vi "create Cell.vi"(8 "error in (no error)":errorcluster, 9 "Column":i32, 10 "Row":i32, 11 "Cell in":refnum<class "Cell.lvclass">) -> (0 "error out":errorcluster, 3 "Cell out":refnum<class "Cell.lvclass">)   [LabVIEW 2019, in "Cell.lvclass"]
uses:
  Cell.lvclass
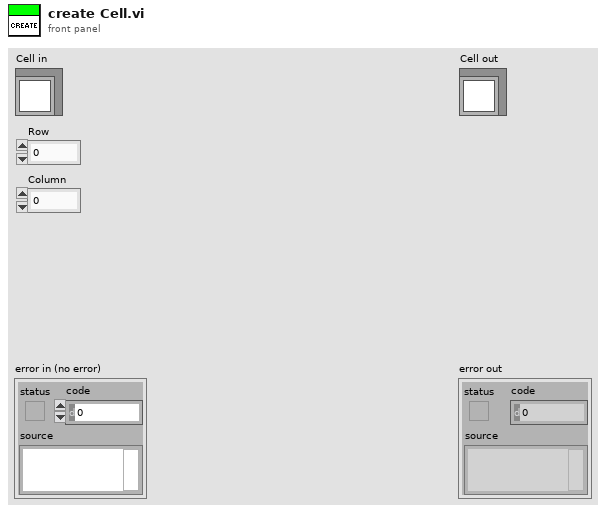
[diagram p1: front panel]
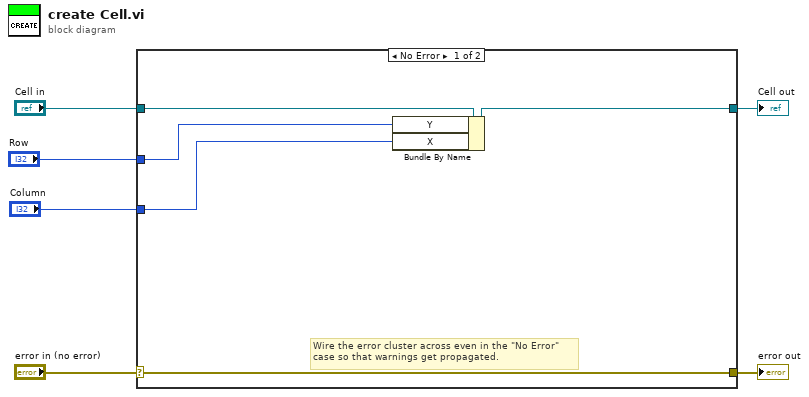
[diagram p0: block diagram]
diagram:
  n1 = case shown="No Error" "error in (no error)" {
    selector: "error in (no error)" -> [w10 w13]
    tunnel: [w10 w13] -> w5
    tunnel: [w9 w12] -> w3
    tunnel: "Cell in" -> [w11 w12]
    tunnel: "Row" -> [w8 _]
    tunnel: "Column" -> [w7 _]
    frame No Error {
      # "Wire the error cluster across even in the \"No Error\"\ncase so that warnings get propagated."
      n2 = Bundle By Name(cluster=w11, "Y"=w8, "X"=w7) -> (w9:refnum<class "Cell.lvclass">)
    }
    frame Error {
    }
  }
  "error out" <- w5
  "Cell out" <- w3
